vi "DirectionToArray.vi"(9 "Posit Array":T1[](array[typedef]), 11 "All Lines":T2) -> (1 "Same Dir as array?":bool)   [LabVIEW 2014]
uses:
  Libraries/Map Data Folder/All-Lines.ctl
  Libraries/Map Data Folder/LineCluster.ctl
  Libraries/Map Data Folder/LineConnection.ctl
  Libraries/Contact Data/Position.ctl
  <vilib>/Analysis/baseanly.llb/Mean (DBL).vi
  Libraries/Map Data Folder/Map Data.lvlib
  <vilib>/Analysis/NI_AALBase.lvlib
  Libraries/Contact Data/Contact Data.lvlib
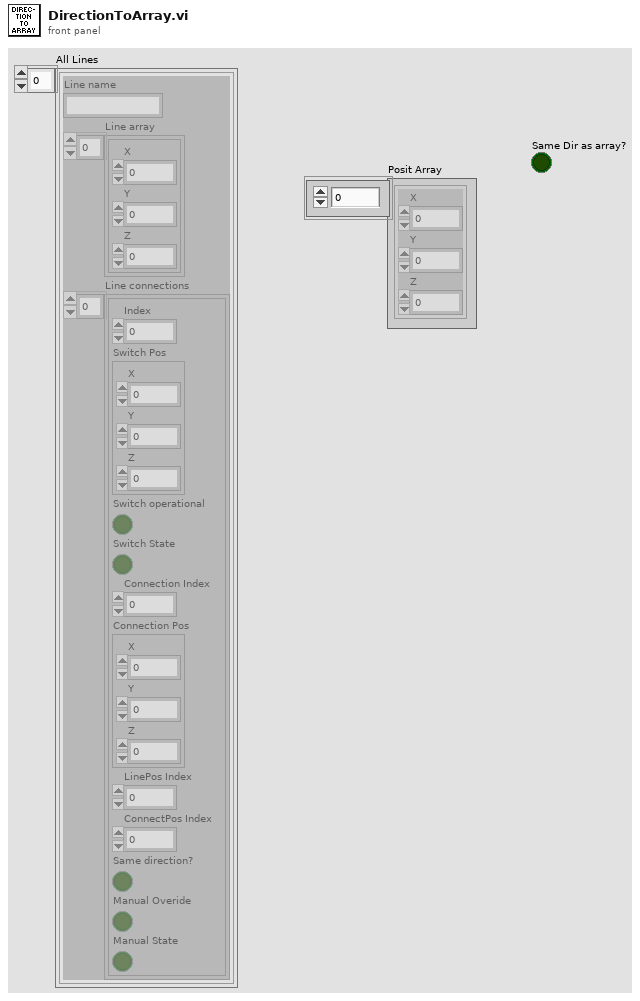
[diagram p1: front panel]
types:
  T1 = typedef "Contact Data.lvlib/Position.ctl" = cluster{"X":dbl, "Y":dbl, "Z":dbl}
  T2 = typedef "Map Data.lvlib/All-Lines.ctl" = T3[]
  T3 = typedef "Map Data.lvlib/LineCluster.ctl" = cluster{"Line name":string, "Line array":cluster{"X":dbl, "Y":dbl, "Z":dbl}[], "Line connections":T4[]}
  T4 = typedef "Map Data.lvlib/LineConnection.ctl" = cluster{"Index":i32, "Switch Pos":cluster{"X":dbl, "Y":dbl, "Z":dbl}, "Switch operational":bool, "Switch State":bool, "Connection Index":i32, "Connection Pos":cluster{"X":dbl, "Y":dbl, "Z":dbl}, "LinePos Index":i32, "ConnectPos Index":i32, "Same direction?":bool, "Manual Overide":bool, "Manual State":bool}
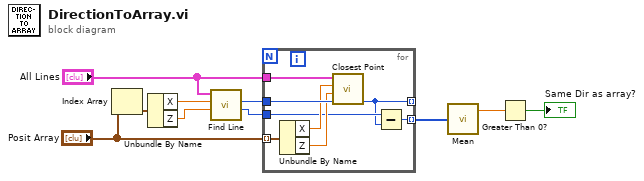
[diagram p0: block diagram]
diagram:
  n1 = Index Array(array="Posit Array") -> (element=w10:T1)  [unwired: 1 in]
  n2 = Unbundle By Name(w10) -> ("X"=w9:dbl, "Z"=w8:dbl)
  n3 = call "Find Line.vi"("Z"=w8, "X"=w9, "All Lines"="All Lines") -> ("Index on Line"=w4:i32, "Nearest Line"=w5:i32)  [unwired: 5 in, 2 out]
  n4 = for {
    tunnel: "Posit Array" -> [w16] mode=indexing
    tunnel: "All Lines" -> [w18]
    tunnel: w5 -> [w17]
    tunnel: [w12] -> _ mode=indexing
    tunnel: w4 -> [w13]
    tunnel: [w11] -> w3 mode=indexing
    n5 = Unbundle By Name(w16) -> ("X"=w15:dbl, "Z"=w14:dbl)
    n6 = call "Closest Point.vi"("index"=w17, "Y in"=w14, "X in"=w15, "All Lines"=w18) -> ("Index on Line"=w12:i32)  [unwired: 5 in, 2 out]
    n7 = Subtract(x=w13, y=w12) -> (x-y=w11:i32)
  }
  n8 = call-poly <vilib>:"Mean.vi"("X"=w3) -> ("mean"=w2:dbl)  [unwired: 1 out]
  n9 = Greater Than 0?(x=w2) -> (x > 0?=→"Same Dir as array?":bool)
